vi "Add Depends Values.vi"(8 "error in (no error)":errorcluster, 9 "Build Type String":string, 10 "Dependencies Set":set{string}(c389), 11 "Map in":map{string, string}(c390)) -> (0 "error out":errorcluster, 3 "Map out":map{string, string}(c390))   [LabVIEW 2019, in "NIPKG Packager.lvclass"]
uses:
  NIPKG Packager.lvclass
  NIPKG Naming/NIPKG Naming.lvlib
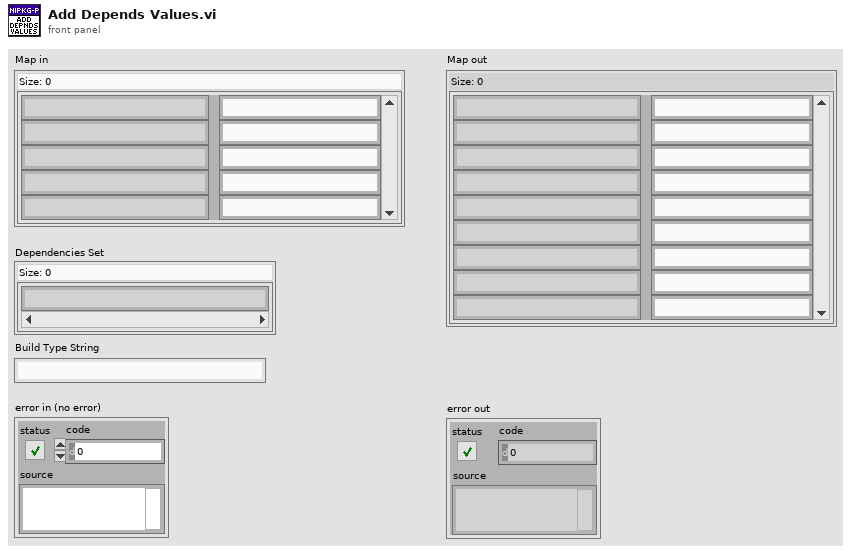
[diagram p1: front panel]
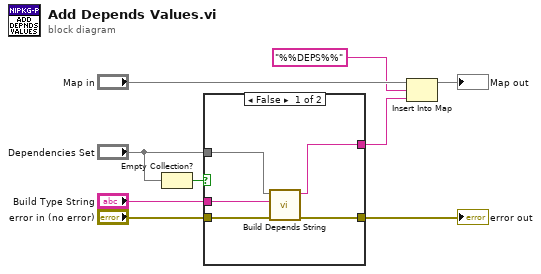
[diagram p0: block diagram]
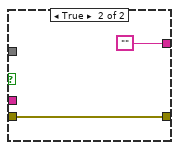
[diagram p2: hidden frame]
diagram:
  n1 = Empty Collection?(1:"Dependencies Set") -> (0:w1:bool)
  n2 = case shown="False" w1 {
    tunnel: [w10 "" ("spreadsheet string")] -> w6
    tunnel: "error in (no error)" -> [w13 w15]
    tunnel: [w11 w15] -> w4
    tunnel: "Build Type String" -> [w12 _]
    tunnel: "Dependencies Set" -> [w14 _]
    frame False {
      n3 = call "Build Depends String.vi"("error in (no error)"=w13, "Build Type String"=w12, "Dependencies Set"=w14) -> ("error out"=w11:errorcluster, "DEPENDS String"=w10:string)  [unwired: 7 in]
    }
    frame True {
    }
  }
  "error out" <- w4
  n4 = Insert Into Map(map in="Map in", key="%%DEPS%%", value=w6) -> (map out=→"Map out":map{string, string})  [unwired: 2 out]
